vi "Define Custom Glyphs by Extension.vi"(8 "error in (no error)":errorcluster, 11 "File Explorer in":refnum<class "File Explorer.lvclass">) -> (0 "error out":errorcluster, 3 "File Explorer out":refnum<class "File Explorer.lvclass">)   [LabVIEW 2017, in "File Explorer.lvlib" / "File Explorer.lvclass"]
uses:
  <vilib>/gpm_packages/@cs/file-explorer-extension/Source/File Explorer/File Explorer/File Explorer.lvclass
  <vilib>/gpm_packages/@cs/file-explorer-extension/Source/File Explorer/File Explorer/Custom Glyph Definition.ctl
  <vilib>/picture/picture.llb/imagedata.ctl
  <vilib>/gpm_packages/@cs/file-explorer-extension/Source/File Explorer/File Explorer/File Explorer.lvclass/File Explorer.ctl
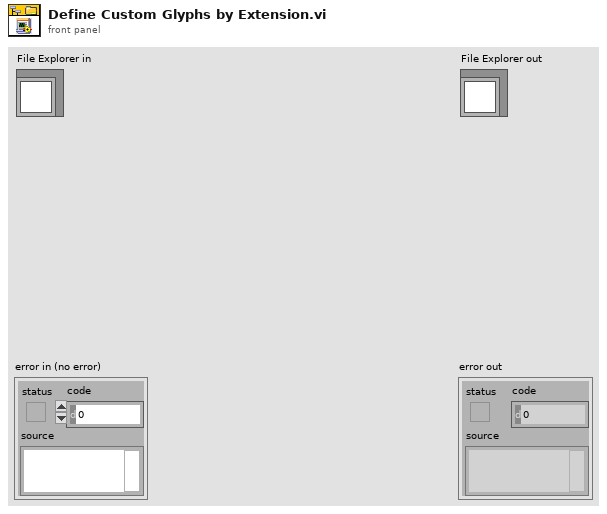
[diagram p1: front panel]
types:
  T1 = typedef "File Explorer.lvlib/File Explorer.lvclass/Custom Glyph Definition.ctl" = cluster{"Extension":string, "Glyph":T2}
  T2 = typedef "imagedata.ctl" = cluster{"image type":i32, "image depth":i32, "image":u8[], "mask":u8[], "colors":u32[], "Rectangle":cluster{"left":i16, "top":i16, "right":i16, "bottom":i16}}
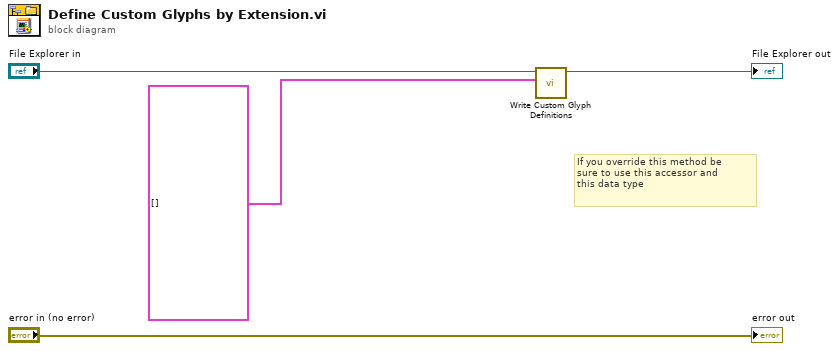
[diagram p0: block diagram]
diagram:
  # "If you override this method be\nsure to use this accessor and \nthis data type"
  n1 = call <vilib>:"Write Custom Glyph Definitions.vi"("Custom Glyph Definitions"=T1[] [], "File Explorer in"="File Explorer in") -> ("File Explorer out"=→"File Explorer out":refnum<class "File Explorer.lvclass">)  [unwired: 9 in]
  "error out" <- "error in (no error)"
